vi "write_bus_header.vi"(8 "Count":u8, 11 "Bus":u8) -> ()   [LabVIEW 2011]
uses:
  <vilib>/rvi/DataTransferAndStorage/Container/Common/niFpgaContainerExecOnDevCompGetState.vi
  <vilib>/rvi/FIFO/Fifo_Resource/nirvififoEmulationSetSize.vi
  <vilib>/rvi/DataTransferAndStorage/Container/Common/niFpgaContainerGetUniqueNameForEmu.vi
  <vilib>/rvi/interface/RandomDataEmulation/nirviRandomDataFPGAFIFO.vi
  <vilib>/rvi/interface/RandomDataEmulation/niFpgaRandomDataHandleErrors.vi
  <vilib>/rvi/eio/common/nirviEmuReportErrorAndStop.vi
  <vilib>/rvi/DataTransferAndStorage/Container/XNode/niFpgaContainer.xnode
  <vilib>/rvi/FIFO/Fifo_Resource/niFpgaFifoEmulationRefIn.vi
panel:
  # "Bus number"
  # "Number of bytes (1..255)"
  # "Write a bus header to the local write FIFO for the demultiplexer."
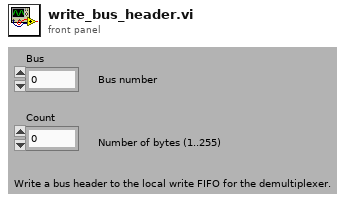
[diagram p1: front panel]
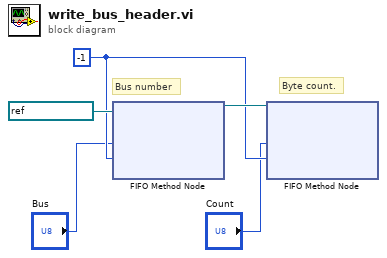
[diagram p0: block diagram]
diagram:
  w3 = -1 ("Timeout")
  # "Byte count."
  # "Bus number"
  n1 = xnode ("FIFO Method Node")("Element"="Bus", "Timeout"=w3, "FIFO In"=refnum<k21> "Local write" ("FIFO")) -> ("FIFO Out"=w4:refnum<k21>)  [unwired: 1 out]
  n2 = xnode ("FIFO Method Node")("Element"="Count", "Timeout"=w3, "FIFO In"=w4) -> ()  [unwired: 2 out]
